vi "Get Struct.vi"(11 "reference":refnum<vi>) -> (2 "Position":T1, 3 "Gen Refnum":refnum<vi>)   [LabVIEW 2015]
uses:
  <vilib>/Utility/miscctls.llb/LVPositionTypeDef.ctl
panel:
  out "Position 2":T1
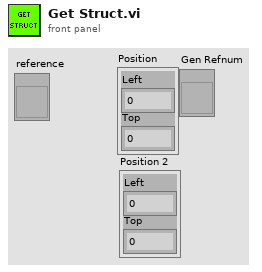
[diagram p1: front panel]
types:
  T1 = typedef "LVPositionTypeDef.ctl" = cluster{"Left":i32, "Top":i32}
  T2 = typedef "LVRectTypeDef.ctl" = cluster{"Left":i16, "Top":i16, "Right":i16, "Bottom":i16}
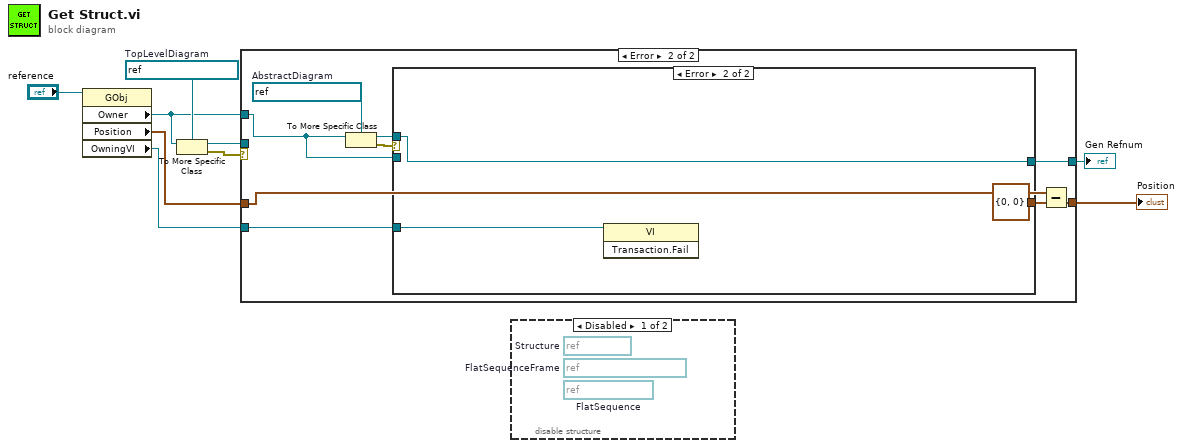
[diagram p0: block diagram]
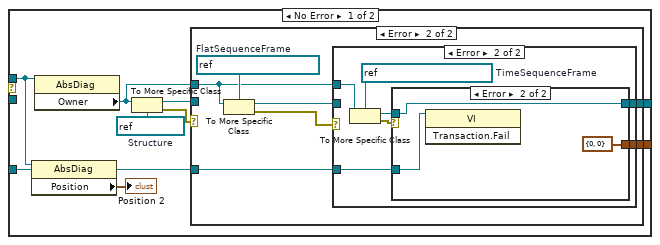
[diagram p4: hidden frame]
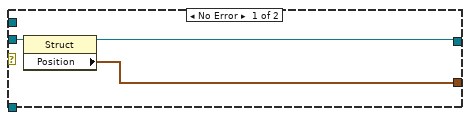
[diagram p5: hidden frame]
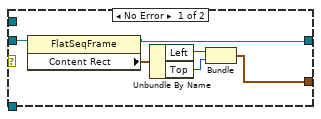
[diagram p6: hidden frame]
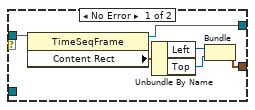
[diagram p7: hidden frame]
diagram:
  w9 = refnum<vi> refnum  # TopLevelDiagram
  n1 = property class="GObj"(reference="reference") -> ("Owner"=w2:refnum<vi>, "Position"=w5:T1, "OwningVI"=w3:refnum<vi>)  [unwired: 1 in, 2 out]
  n2 = To More Specific Class(target class=w9, reference=w2) -> (specific class reference=w6:refnum<vi>, error out=w8:errorcluster)  [unwired: 1 in]
  n3 = case shown="Error" w8 {
    tunnel: [w11 w13] -> w1
    tunnel: w5 -> [w11 w12]
    tunnel: [w10 w19] -> w4
    tunnel: w6 -> [w10 _]
    tunnel: w2 -> [_ w15]
    tunnel: w3 -> [_ w17]
    frame No Error {
    }
    frame Error {
      w20 = refnum<vi> refnum  # AbstractDiagram
      n4 = To More Specific Class(target class=w20, reference=w15) -> (specific class reference=w16:refnum<vi>, error out=w18:errorcluster)  [unwired: 1 in]
      n5 = case shown="Error" w18 {
        tunnel: [w27 T1 {"Left"=0, "Top"=0} ("Position")] -> w14
        tunnel: [w26 w64] -> w19
        tunnel: w16 -> [w22 w64]
        tunnel: w17 -> [w24 w63]
        tunnel: w15 -> [_ _]
        frame No Error {
          w29 = refnum<vi> refnum  # Structure
          n6 = property class="AbsDiag"(reference=w22) -> ("Position"=→"Position 2":T1)  [unwired: 1 in, 2 out]
          n7 = property class="AbsDiag"(reference=w22) -> ("Owner"=w23:refnum<vi>)  [unwired: 1 in, 2 out]
          n8 = To More Specific Class(target class=w29, reference=w23) -> (specific class reference=w28:refnum<vi>, error out=w25:errorcluster)  [unwired: 1 in]
          n9 = case shown="Error" w25 {
            tunnel: w28 -> [w32 _]
            tunnel: [w30 w36] -> w27
            tunnel: [w31 w37] -> w26
            tunnel: w23 -> [_ w33]
            tunnel: w24 -> [_ w34]
            frame No Error {
              n10 = property class="Struct"(reference=w32) -> (reference out=w31:refnum<vi>, "Position"=w30:T1)  [unwired: 1 in, 1 out]
            }
            frame Error {
              w39 = refnum<vi> refnum  # FlatSequenceFrame
              n11 = To More Specific Class(target class=w39, reference=w33) -> (specific class reference=w38:refnum<vi>, error out=w35:errorcluster)  [unwired: 1 in]
              n12 = case shown="Error" w35 {
                tunnel: w38 -> [w42 _]
                tunnel: [w41 w50] -> w37
                tunnel: [w40 w47] -> w36
                tunnel: w33 -> [_ w52]
                tunnel: w34 -> [_ w46]
                frame No Error {
                  n13 = property class="FlatSeqFrame"(reference=w42) -> (reference out=w41:refnum<vi>, "Content Rect"=w43:T2)  [unwired: 1 in, 1 out]
                  n14 = Unbundle By Name(w43) -> ("Left"=w44:i16, "Top"=w45:i16)
                  n15 = Bundle("Left"=w44, "Top"=w45) -> (w40:cluster{"Left":i16, "Top":i16})  [unwired: 1 in]
                }
                frame Error {
                  w51 = refnum<vi> refnum  # TimeSequenceFrame
                  n16 = To More Specific Class(target class=w51, reference=w52) -> (specific class reference=w49:refnum<vi>, error out=w48:errorcluster)  [unwired: 1 in]
                  n17 = case shown="Error" w48 {
                    tunnel: [w53 w61] -> w50
                    tunnel: w49 -> [w55 w61]
                    tunnel: [w54 cluster{"Left":i16, "Top":i16} {"Left"=0, "Top"=0}] -> w47
                    tunnel: w46 -> [_ w60]
                    frame No Error {
                      n18 = property class="TimeSeqFrame"(reference=w55) -> (reference out=w53:refnum<vi>, "Content Rect"=w58:T2)  [unwired: 1 in, 1 out]
                      n19 = Unbundle By Name(w58) -> ("Left"=w57:i16, "Top"=w56:i16)
                      n20 = Bundle("Left"=w57, "Top"=w56) -> (w54:cluster{"Left":i16, "Top":i16})  [unwired: 1 in]
                    }
                    frame Error {
                      n21 = invoke class="VI" method="Transaction.Fail"(reference=w60) -> ()  [unwired: 2 in, 3 out]
                    }
                  }
                }
              }
            }
          }
        }
        frame Error {
          n22 = invoke class="VI" method="Transaction.Fail"(reference=w63) -> ()  [unwired: 2 in, 3 out]
        }
      }
      n23 = Subtract(x=w12, y=w14) -> (x-y=w13:T1)
    }
  }
  "Position" <- w1
  "Gen Refnum" <- w4
  n24 = disable-structure shown="Disabled" {
    frame Disabled {
      (unwired) refnum<vi> refnum  # Structure
      (unwired) refnum<vi> refnum  # FlatSequence
      (unwired) refnum<vi> refnum  # FlatSequenceFrame
    }
    frame Enabled {
    }
  }
